vi "Get Gas Output.vi"(8 "error in":errorcluster, 11 "Owlstone OVG-4 in":refnum<class "Owlstone GEN-SYS.lvclass">) -> (0 "error out":errorcluster, 2 "Output":T1 {"Relative Humidity (%)" format="%#.4g"; "Flow Rate (ml/min)" format="%#.0f"; "Concentration (ppm)" format="%#.2g"}, 3 "Owlstone OVG-4 out":refnum<class "Owlstone GEN-SYS.lvclass">)   [LabVIEW 2011, in "Owlstone GEN-SYS.lvclass"]
uses:
  Owlstone GEN-SYS.lvclass
  Vapour Generator/Gas Output.ctl
  Owlstone GEN-SYS.lvclass/Owlstone GEN-SYS.ctl
  Michell Easidew/Michell Easidew.lvclass
  Vapour Generator/Vapour Generator.lvclass
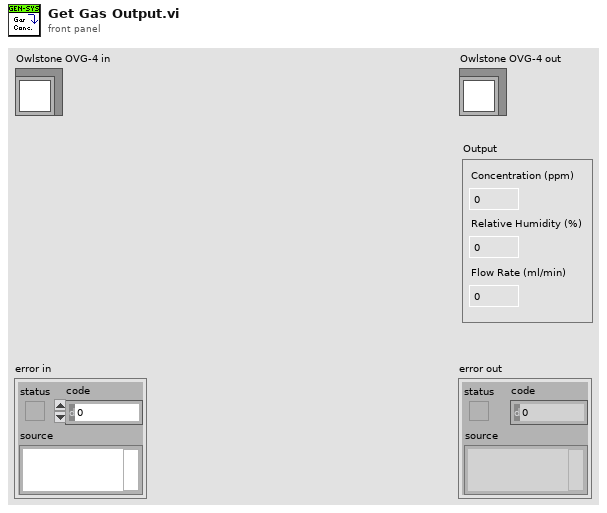
[diagram p1: front panel]
types:
  T1 = typedef "Vapour Generator.lvclass/Gas Output.ctl" = cluster{"Concentration (ppm)":dbl, "Flow Rate (ml/min)":dbl, "Relative Humidity (%)":dbl}
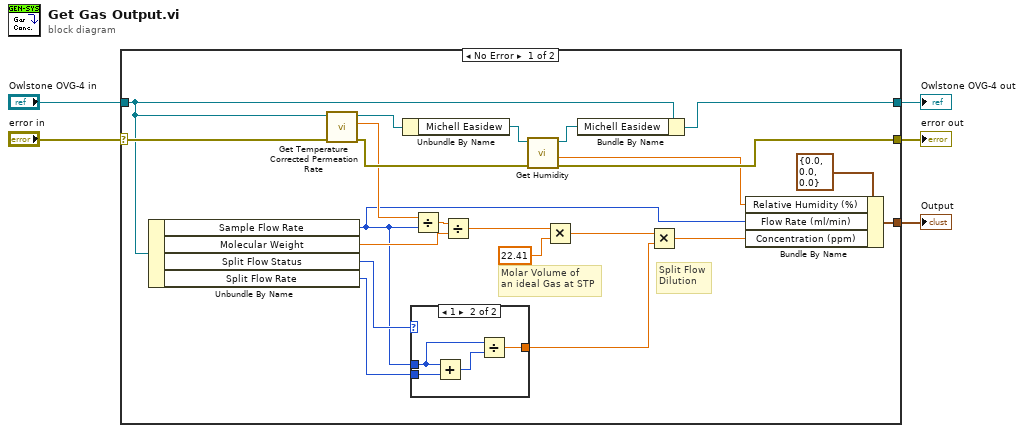
[diagram p0: block diagram]
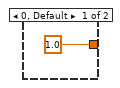
[diagram p2: hidden frame]
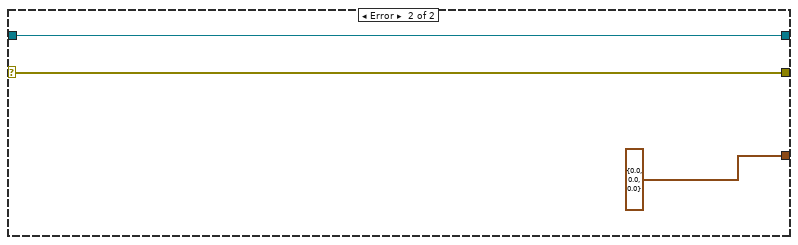
[diagram p3: hidden frame]
diagram:
  n1 = case shown="No Error" "error in" {
    selector: "error in" -> [w14 w35]
    tunnel: [w21 w35] -> w4
    tunnel: [w7 w34] -> w2
    tunnel: "Owlstone OVG-4 in" -> [w8 w34]
    tunnel: [w27 T1 {"Concentration (ppm)"=0.0, "Flow Rate (ml/min)"=0.0, "Relative Humidity (%)"=0.0} ("Output")] -> w1
    frame No Error {
      # "Split Flow\nDilution"
      # "Molar Volume of \nan ideal Gas at STP"
      n2 = Unbundle By Name(w8) -> ("Sample Flow Rate"=w9:i32, "Molecular Weight"=w25:dbl, "Split Flow Status"=w19:u16, "Split Flow Rate"=w18:i32)
      n3 = call-dynamic "Get Temperature Corrected Permeation Rate.vi"("error in"=w14, "Owlstone GEN-SYS in"=w8) -> ("error out"=w11:errorcluster, "Permeation Rate"=w10:dbl, "Owlstone GEN-SYS out"=w13:refnum<class "Owlstone GEN-SYS.lvclass">)  [unwired: 7 in]
      n4 = Unbundle By Name(w13) -> ("Michell Easidew"=w12:refnum<class "Michell Easidew.lvclass">)
      n5 = case shown="1" w19 {
        tunnel: w9 -> [_ w30]
        tunnel: w18 -> [_ w32]
        tunnel: [1.0 w29] -> w16
        frame 0, Default {
        }
        frame 1 {
          n6 = Add(x=w30, y=w32) -> (x+y=w31:i32)
          n7 = Divide(x=w30, y=w31) -> (x/y=w29:dbl)
        }
      }
      n8 = Divide(x=w10, y=w9) -> (x/y=w26:dbl)
      n9 = Divide(x=w26, y=w25) -> (x/y=w24:dbl)
      n10 = call-dynamic "Get Humidity.vi"("error in"=w11, "Michell Easydew in"=w12) -> ("error out"=w21:errorcluster, "Relative Humidity"=w6:dbl, "Michell Easydew out"=w22:refnum<class "Michell Easidew.lvclass">)  [unwired: 4 in, 3 out]
      n11 = Multiply(x=w24, y=22.41) -> (x*y=w17:dbl)
      n12 = Bundle By Name(cluster=w8, "Michell Easidew"=w22) -> (w7:refnum<class "Owlstone GEN-SYS.lvclass">)
      n13 = Multiply(x=w17, y=w16) -> (x*y=w15:dbl)
      n14 = Bundle By Name(cluster=T1 {"Concentration (ppm)"=0.0, "Flow Rate (ml/min)"=0.0, "Relative Humidity (%)"=0.0} ("Output"), "Relative Humidity (%)"=w6, "Flow Rate (ml/min)"=w9, "Concentration (ppm)"=w15) -> (w27:T1)
    }
    frame Error {
    }
  }
  "error out" <- w4
  "Owlstone OVG-4 out" <- w2
  "Output" <- w1
